vi "HuStrategy.vi"(9 "TargetTile":u16(ring)=36, 10 "Hand":u16[](array[ring])) -> (2 "Hu?":bool)   [LabVIEW 2025]
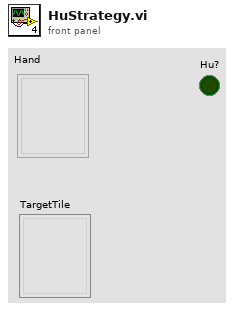
[diagram p1: front panel]
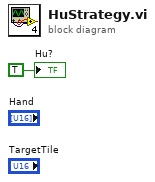
[diagram p0: block diagram]
diagram:
  "Hu?" <- TRUE
